vi "Leitura_pressão2CAN_temperatura.vi"() -> ()   [LabVIEW 2019]
uses:
  <vilib>/Analysis/baseanly.llb/Mean (DBL).vi
  <vilib>/Analysis/NI_AALBase.lvlib
panel:
  out "Derivada":waveform(dbl)[](graph)
  out "Tempo s":dbl
  out "Stop Press 2":bool
  in  "WindowMean":i32=20
  out "Comp Suc":sgl
  out "Error out":errorcluster {"code" format="%.0x"}
  out "Valvula Suc":sgl
  out "error out":errorcluster
  out "XY Graph 2":cluster{dbl[], dbl[]}[](graph)
  out "Stop Press":bool
  out "Stop Temp":bool
  in  "stop":bool
  out "Zerar Temp":bool
  out "Zerar Press":bool
  in  "Zerar":bool
  out "Corpo [ºC]":dbl
  out "Descarga [ºC]":dbl
  out "Reservatório [ºC]":dbl
  out "Sucção [ºC]":dbl
  out "Intermed":dbl format="%0.4f"
  out "Descarga A0":dbl format="%0.4f"
  out "Sucção A1":dbl format="%0.4f"
  out "XY Graph":cluster{dbl[], dbl[]}[](graph)
  out "Descarga/Sucção":dbl
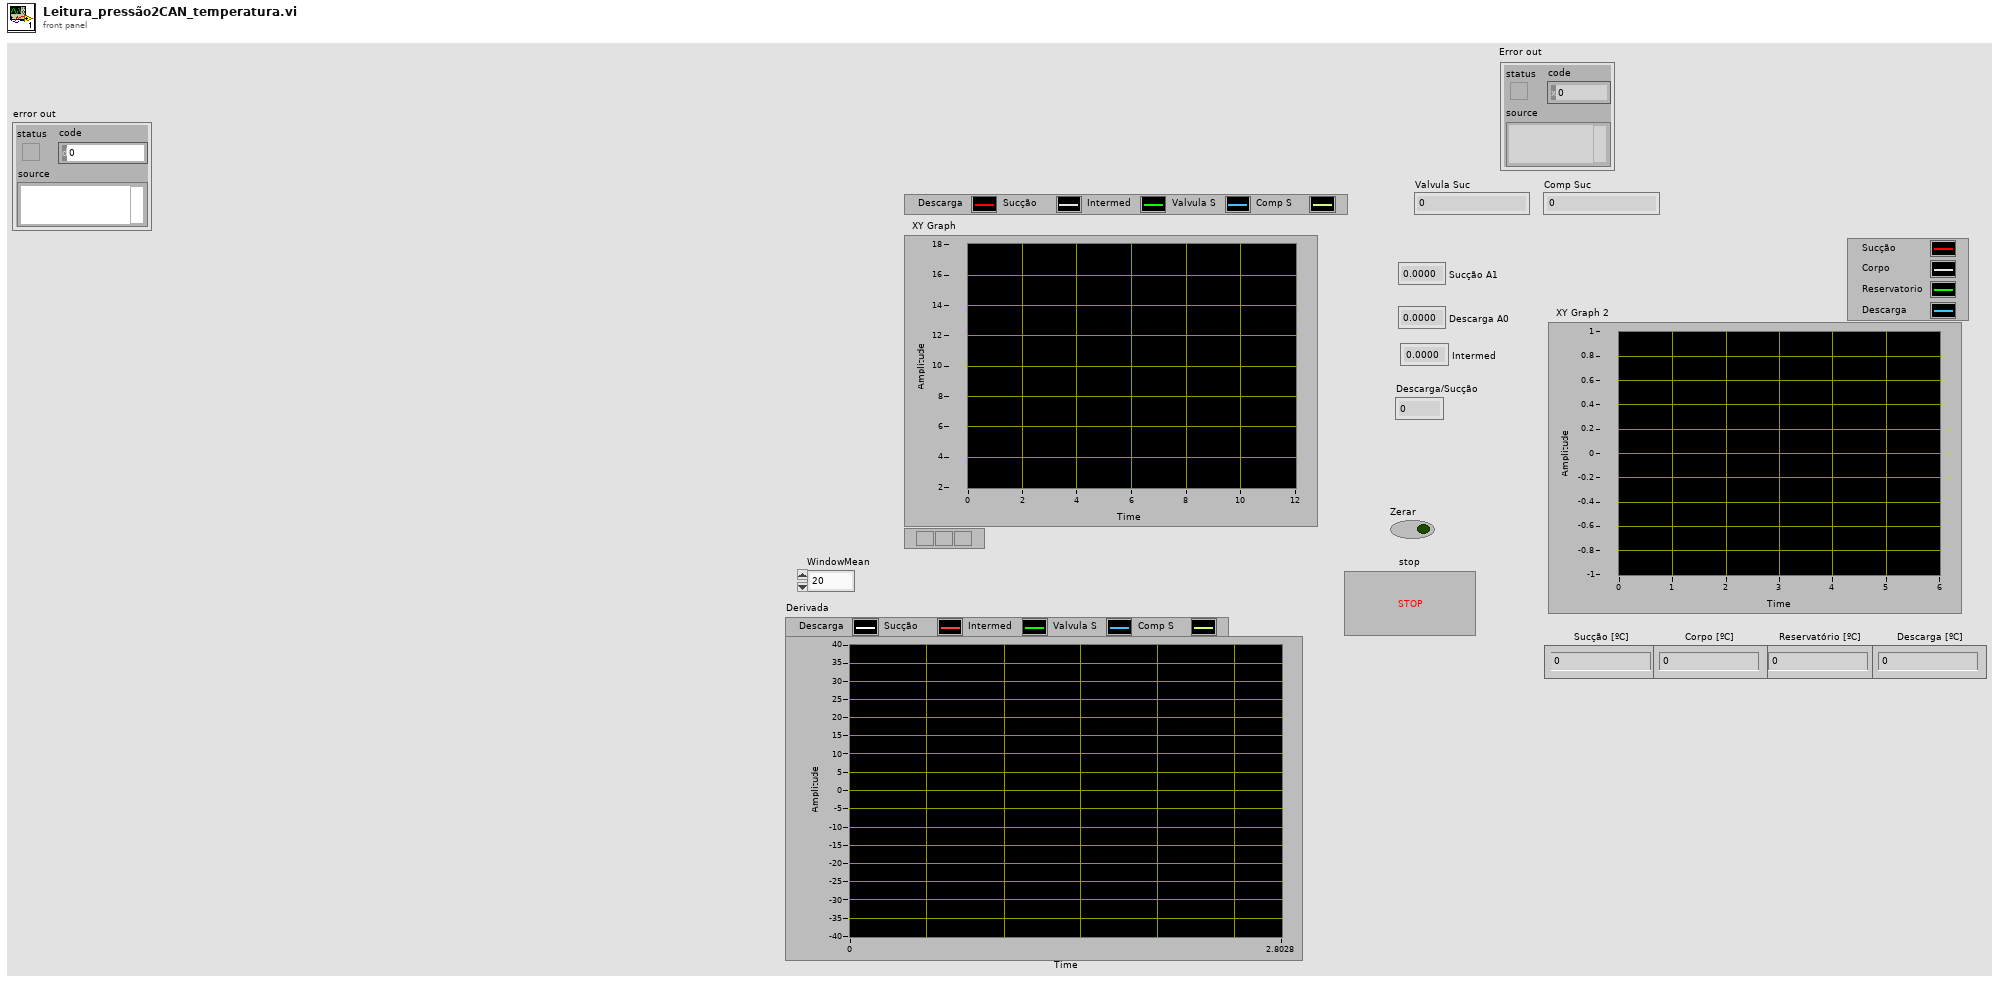
[diagram p1: front panel]
types:
  T1 = enum16{"start remote node", "stop remote node", "reset node", "reset communication", "enter preoperational"}
  T2 = typedef "xobjhandle.ctl" = u32
  T3 = enum16{"big-endian, network order", "native, host order", "little-endian"}
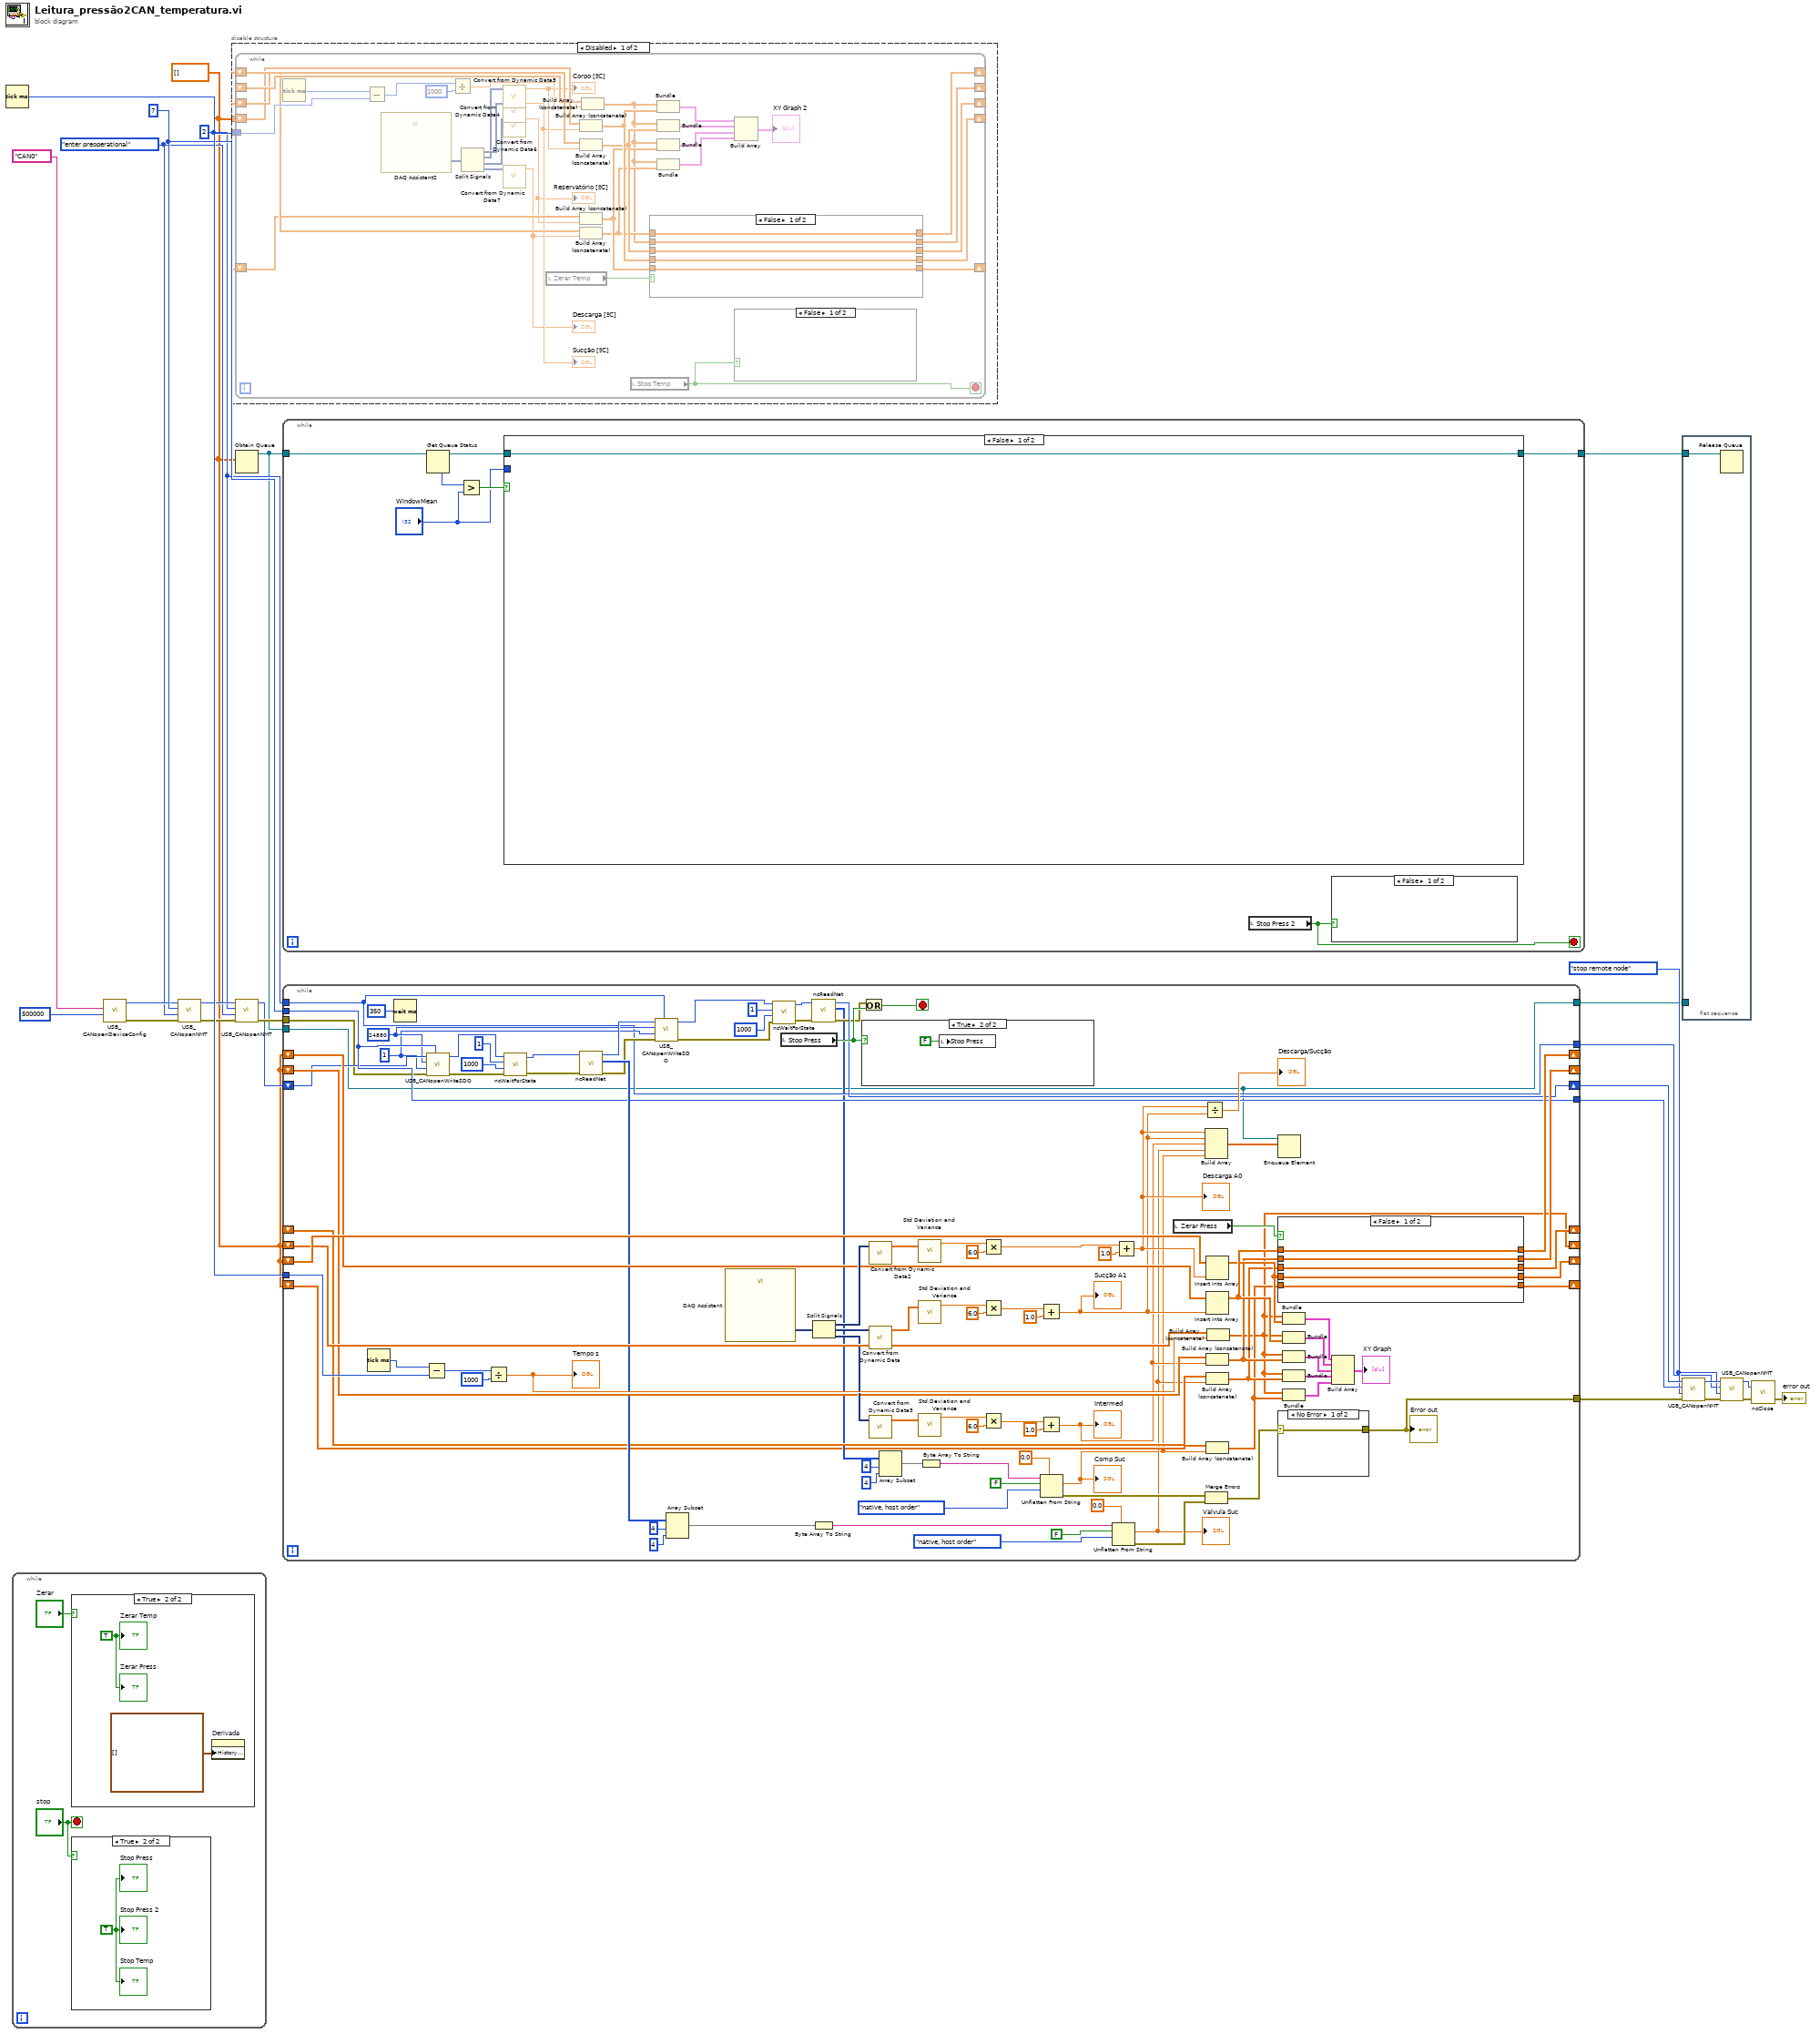
[diagram p0: block diagram]
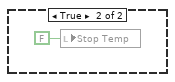
[diagram p2: hidden frame]
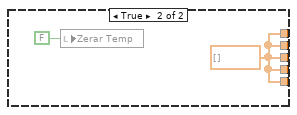
[diagram p3: hidden frame]
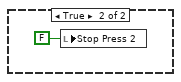
[diagram p5: hidden frame]
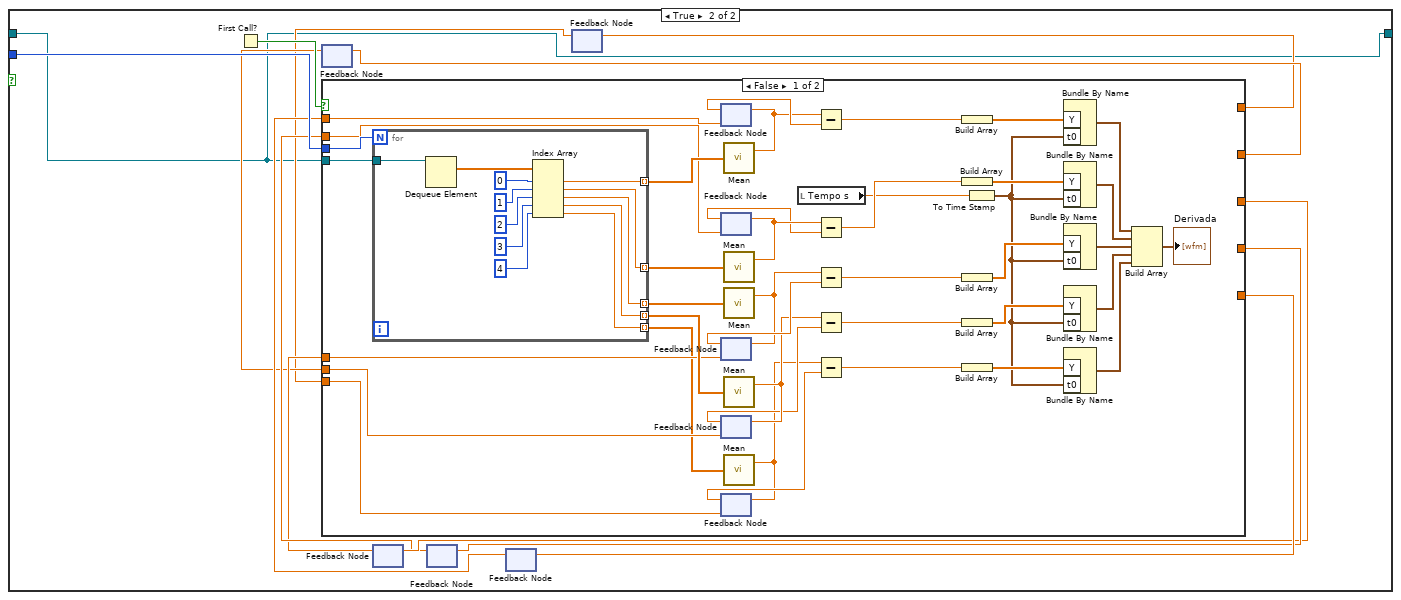
[diagram p6: hidden frame]
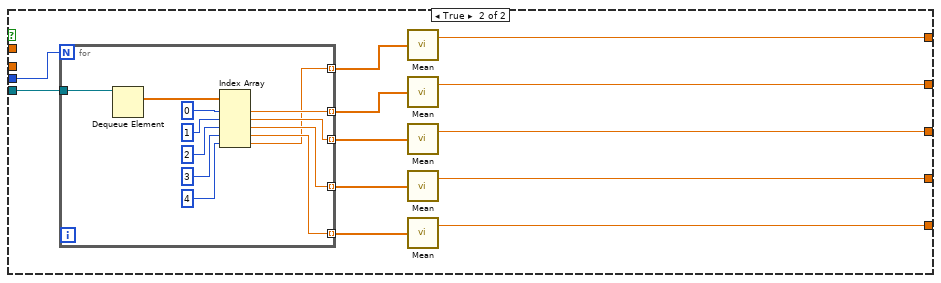
[diagram p7: hidden frame]
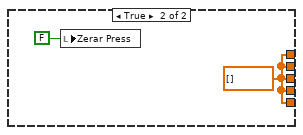
[diagram p12: hidden frame]
diagram:
  w11 = 2
  w12 = T1."enter preoperational" ("Mode")
  w21 = u32 7 ("milliseconds to wait")
  w6 = T1."stop remote node" ("Mode")
  w5 = dbl[] []
  n1 = Tick Count (ms)() -> (millisecond timer value=w26:u32)
  n2 = while {
    stop <- "stop" stop-if-true
    n3 = case shown="True" "Zerar" {
      frame False {
      }
      frame True {
        w31 = TRUE
        n4 = property on="Derivada" class="WFChart (strict)"("History Data"=waveform(dbl)[][] []) -> ()  [unwired: 2 in, 2 out]
        "Zerar Press" <- w31
        "Zerar Temp" <- w31
      }
    }
    n5 = case shown="True" "stop" {
      frame False {
      }
      frame True {
        w29 = TRUE
        "Stop Press" <- w29
        "Stop Temp" <- w29
        "Stop Press 2" <- w29
      }
    }
  }
  n6 = call "USB_CANopenDeviceConfig.vi"("Baudrate"=u32 500000, "Interface"="CAN0") -> ("Error out"=w18:errorcluster, "ObjHandle out"=w17:T2)  [unwired: 8 in]
  n7 = call "USB_CANopenNMT.vi"("error in"=w18, "Mode"=w12, "Node ID"=w21, "ObjHandle in"=w17) -> ("error out"=w15:errorcluster, "ObjHandle out"=w16:T2)  [unwired: 2 in]
  n8 = disable-structure shown="Disabled" {
    disable-tunnel: w26 -> [w33 _]
    disable-tunnel: w5 -> [w32 _]
    frame Disabled {
      n9 = while {
        tunnel: w33 -> [w62]
        shift-right: [w51] -> _
        shift-left: w32 -> [w50]
        shift-right: [w53] -> _
        shift-left: w32 -> [w52]
        shift-right: [w55] -> _
        shift-left: w32 -> [w54]
        shift-right: [w57] -> _
        shift-left: w32 -> [w56]
        shift-right: [w58] -> _
        shift-left: _ -> [w60]
        stop <- w39 stop-if-true
        n10 = Tick Count (ms)() -> (millisecond timer value=w63:u32)
        n11 = Subtract(x=w63, y=w62) -> (x-y=w64:u32)
        n12 = call "DAQ Assistant2"() -> ("data"=w69:dynamicdata)  [unwired: 17 in, 2 out]
        n13 = Divide(x=w64, y=u32 1000) -> (x/y=w59:dbl)
        n14 = Split Signals(w69) -> (w68:dynamicdata, w67:dynamicdata, w66:dynamicdata, w65:dynamicdata)  [unwired: 4 in]
        n15 = call "Convert from Dynamic Data5"("Dynamic Data Type"=w67) -> ("Scalar"=w48:dbl)  [unwired: 3 in]
        "Corpo [ºC]" <- w48
        n16 = call "Convert from Dynamic Data4"("Dynamic Data Type"=w68) -> ("Scalar"=w49:dbl)  [unwired: 3 in]
        "Sucção [ºC]" <- w49
        n17 = call "Convert from Dynamic Data6"("Dynamic Data Type"=w66) -> ("Scalar"=w47:dbl)  [unwired: 3 in]
        "Reservatório [ºC]" <- w47
        n18 = call "Convert from Dynamic Data7"("Dynamic Data Type"=w65) -> ("Scalar"=w46:dbl)  [unwired: 3 in]
        "Descarga [ºC]" <- w46
        n19 = local read "Zerar Temp"() -> (w40:bool)
        n20 = Build Array (concatenate)(w50, w49) -> (w45:dbl[])
        n21 = Build Array (concatenate)(w52, w48) -> (w44:dbl[])
        n22 = Build Array (concatenate)(w54, w47) -> (w43:dbl[])
        n23 = Build Array (concatenate)(w56, w46) -> (w42:dbl[])
        n24 = Build Array (concatenate)(w60, w59) -> (w41:dbl[])
        n25 = local read "Stop Temp"() -> (w39:bool)
        n26 = case shown="False" w40 {
          tunnel: w41 -> [w75 _]
          tunnel: [w75 w76] -> w58
          tunnel: w42 -> [w74 _]
          tunnel: [w74 w76] -> w57
          tunnel: w43 -> [w73 _]
          tunnel: [w73 w76] -> w55
          tunnel: w44 -> [w72 _]
          tunnel: [w72 w76] -> w53
          tunnel: w45 -> [w71 _]
          tunnel: [w71 w76] -> w51
          frame False {
          }
          frame True {
            w76 = dbl[] []
            n27 = local write "Zerar Temp"(FALSE ("Zerar Temp")) -> ()
          }
        }
        n28 = Bundle(w41, w45) -> (w37:cluster{dbl[], dbl[]})  [unwired: 1 in]
        n29 = Bundle(w41, w44) -> (w36:cluster{dbl[], dbl[]})  [unwired: 1 in]
        n30 = Bundle(w41, w43) -> (w35:cluster{dbl[], dbl[]})  [unwired: 1 in]
        n31 = Bundle(w41, w42) -> (w34:cluster{dbl[], dbl[]})  [unwired: 1 in]
        n32 = Build Array(w37, w36, w35, w34) -> (→"XY Graph 2":cluster{dbl[], dbl[]}[])
        n33 = case shown="False" w39 {
          frame False {
          }
          frame True {
            n34 = local write "Stop Temp"(FALSE ("Stop Temp")) -> ()
          }
        }
      }
    }
    frame Enabled {
    }
  }
  n35 = Obtain Queue(element data type=w5) -> (queue out=w4:refnum<queue>)  [unwired: 4 in, 2 out]
  n36 = call "USB_CANopenNMT.vi"("error in"=w15, "Mode"=w12, "Node ID"=w11, "ObjHandle in"=w16) -> ("error out"=w14:errorcluster, "ObjHandle out"=w13:T2)  [unwired: 2 in]
  n37 = while {
    tunnel: w4 -> [w84]
    tunnel: [w78] -> w3
    stop <- w79 stop-if-true
    n38 = Get Queue Status(queue=w84) -> (queue out=w80:refnum<queue>, # elements in queue=w83:i32)  [unwired: 2 in, 6 out]
    n39 = Greater?(x=w83, y="WindowMean") -> (0:w82:bool)
    n40 = case shown="False" w82 {
      tunnel: "WindowMean" -> [_ w99]
      tunnel: w80 -> [w86 w87]
      tunnel: [w86 w87] -> w78
      frame False {
      }
      frame True {
        n41 = First Call?() -> (First Call?: T/F=w98:bool)
        n42 = feedback #1() -> (w90:dbl)  [unwired: 1 in]
        n43 = feedback #2() -> (w91:dbl)  [unwired: 1 in]
        n44 = feedback #3() -> (w92:dbl)  [unwired: 1 in]
        n45 = feedback #4() -> (w93:dbl)  [unwired: 1 in]
        n46 = feedback #5() -> (w88:dbl)  [unwired: 1 in]
        n47 = case shown="False" w98 {
          tunnel: w99 -> [w139 w154]
          tunnel: w87 -> [w138 w159]
          tunnel: [_ w158] -> w94
          tunnel: [_ w157] -> w95
          tunnel: [_ w156] -> w96
          tunnel: [_ w155] -> w97
          tunnel: w93 -> [w125 _]
          tunnel: w92 -> [w124 _]
          tunnel: w91 -> [w123 _]
          tunnel: w90 -> [w122 _]
          tunnel: [_ w152] -> w89
          tunnel: w88 -> [w118 _]
          frame False {
            n48 = for {
              N: w139 -> [_]
              tunnel: w138 -> [w151]
              tunnel: [w145] -> w135 mode=indexing
              tunnel: [w144] -> w128 mode=indexing
              tunnel: [w143] -> w127 mode=indexing
              tunnel: [w142] -> w126 mode=indexing
              tunnel: [w140] -> w119 mode=indexing
              n49 = Dequeue Element(queue=w151) -> (element=w150:dbl[])  [unwired: 2 in, 3 out]
              n50 = Index Array(array=w150, index #1=0 ("index"), index #2=1 ("index"), index #3=2 ("index"), index #4=3 ("index"), index #5=4 ("index")) -> (element #1=w145:dbl, element #2=w144:dbl, element #3=w143:dbl, element #4=w142:dbl, element #5=w140:dbl)
            }
            n51 = feedback #6(w125) -> (w137:dbl)
            n52 = feedback #7(w124) -> (w133:dbl)
            n53 = feedback #8(w123) -> (w132:dbl)
            n54 = feedback #9(w122) -> (w129:dbl)
            n55 = feedback #10(w118) -> (w121:dbl)
            n56 = call-poly <vilib>:"Mean.vi"("X"=w135) -> ("mean"=w136:dbl)  [unwired: 1 out]
            n57 = feedback-in #6(w136) -> ()
            n58 = call-poly <vilib>:"Mean.vi"("X"=w128) -> ("mean"=w134:dbl)  [unwired: 1 out]
            n59 = feedback-in #7(w134) -> ()
            n60 = call-poly <vilib>:"Mean.vi"("X"=w127) -> ("mean"=w131:dbl)  [unwired: 1 out]
            n61 = feedback-in #8(w131) -> ()
            n62 = call-poly <vilib>:"Mean.vi"("X"=w126) -> ("mean"=w130:dbl)  [unwired: 1 out]
            n63 = feedback-in #9(w130) -> ()
            n64 = call-poly <vilib>:"Mean.vi"("X"=w119) -> ("mean"=w120:dbl)  [unwired: 1 out]
            n65 = feedback-in #10(w120) -> ()
            n66 = local read "Tempo s"() -> (w102:dbl)
            n67 = Subtract(x=w136, y=w137) -> (x-y=w116:dbl)
            n68 = Subtract(x=w134, y=w133) -> (x-y=w115:dbl)
            n69 = Subtract(x=w131, y=w132) -> (x-y=w114:dbl)
            n70 = Subtract(x=w130, y=w129) -> (x-y=w113:dbl)
            n71 = Subtract(x=w120, y=w121) -> (x-y=w112:dbl)
            n72 = Build Array(w116) -> (w117:dbl[])
            n73 = Build Array(w115) -> (w111:dbl[])
            n74 = Build Array(w114) -> (w110:dbl[])
            n75 = Build Array(w113) -> (w109:dbl[])
            n76 = Build Array(w112) -> (w108:dbl[])
            n77 = To Time Stamp(1:w102) -> (0:w101:timestamp)
            n78 = Bundle By Name("Y"=w117, "t0"=w101) -> (w107:waveform(dbl))  [unwired: 1 in]
            n79 = Bundle By Name("Y"=w111, "t0"=w101) -> (w106:waveform(dbl))  [unwired: 1 in]
            n80 = Bundle By Name("Y"=w110, "t0"=w101) -> (w105:waveform(dbl))  [unwired: 1 in]
            n81 = Bundle By Name("Y"=w109, "t0"=w101) -> (w104:waveform(dbl))  [unwired: 1 in]
            n82 = Bundle By Name("Y"=w108, "t0"=w101) -> (w103:waveform(dbl))  [unwired: 1 in]
            n83 = Build Array(w107, w106, w105, w104, w103) -> (→"Derivada":waveform(dbl)[])
          }
          frame True {
            n84 = for {
              N: w154 -> [_]
              tunnel: w159 -> [w175]
              tunnel: [w169] -> w160 mode=indexing
              tunnel: [w168] -> w161 mode=indexing
              tunnel: [w167] -> w162 mode=indexing
              tunnel: [w166] -> w163 mode=indexing
              tunnel: [w164] -> w153 mode=indexing
              n85 = Dequeue Element(queue=w175) -> (element=w174:dbl[])  [unwired: 2 in, 3 out]
              n86 = Index Array(array=w174, index #1=0 ("index"), index #2=1 ("index"), index #3=2 ("index"), index #4=3 ("index"), index #5=4 ("index")) -> (element #1=w169:dbl, element #2=w168:dbl, element #3=w167:dbl, element #4=w166:dbl, element #5=w164:dbl)
            }
            n87 = call-poly <vilib>:"Mean.vi"("X"=w153) -> ("mean"=w152:dbl)  [unwired: 1 out]
            n88 = call-poly <vilib>:"Mean.vi"("X"=w160) -> ("mean"=w158:dbl)  [unwired: 1 out]
            n89 = call-poly <vilib>:"Mean.vi"("X"=w161) -> ("mean"=w157:dbl)  [unwired: 1 out]
            n90 = call-poly <vilib>:"Mean.vi"("X"=w162) -> ("mean"=w156:dbl)  [unwired: 1 out]
            n91 = call-poly <vilib>:"Mean.vi"("X"=w163) -> ("mean"=w155:dbl)  [unwired: 1 out]
          }
        }
        n92 = feedback-in #1(w94) -> ()
        n93 = feedback-in #2(w95) -> ()
        n94 = feedback-in #3(w96) -> ()
        n95 = feedback-in #4(w97) -> ()
        n96 = feedback-in #5(w89) -> ()
      }
    }
    n97 = local read "Stop Press 2"() -> (w79:bool)
    n98 = case shown="False" w79 {
      frame False {
      }
      frame True {
        n99 = local write "Stop Press 2"(FALSE ("Stop Press")) -> ()
      }
    }
  }
  n100 = while {
    shift-right: [w263] -> _
    shift-left: w5 -> [w271]
    shift-right: [w264] -> _
    shift-left: w5 -> [w270]
    shift-right: [w183] -> _
    shift-left: w5 -> [w256]
    tunnel: w26 -> [w247]
    shift-right: [w237] -> _
    shift-left: w5 -> [w239]
    tunnel: [w226] -> w24
    tunnel: [w227] -> w23
    tunnel: w21 -> [w227]
    shift-right: [w201] -> w22
    shift-left: w13 -> [w219]
    tunnel: w14 -> [w218]
    shift-right: [w214] -> _
    shift-left: _ -> [w217]
    tunnel: w11 -> [w200]
    tunnel: [w200] -> w2
    shift-right: [w184] -> _
    shift-left: w5 -> [w187]
    tunnel: w4 -> [w176]
    tunnel: [w176] -> w1
    stop <- w204 stop-if-true
    w202 = u8 1 ("Sub Index")
    w203 = u16 24880 ("Index")
    n101 = Tick Count (ms)() -> (millisecond timer value=w249:u32)
    n102 = Wait (ms)(milliseconds to wait=u32 350) -> ()  [unwired: 1 out]
    n103 = Subtract(x=w249, y=w247) -> (x-y=w248:u32)
    n104 = call "USB_CANopenWriteSDO.vi"("Node ID"=w227, "error in"=w218, "Sub Index"=w202, "Index"=w203, "ObjHandle in"=w219) -> ("error out"=w221:errorcluster, "ObjHandle out"=w223:T2)  [unwired: 5 in]
    n105 = Divide(x=w248, y=u32 1000) -> (x/y=w250:dbl)
    "Tempo s" <- w250
    n106 = call <vilib>:"ncWaitForState.vi"("Error in"=w221, "Timeout"=u32 1000, "DesiredState"=u32 1, "ObjHandle in"=w223) -> ("Error out"=w220:errorcluster, "ObjHandle out"=w222:T2)  [unwired: 1 out]
    n107 = call <vilib>:"ncReadNet.vi"("ObjHandle in"=w222, "Error in"=w220) -> ("ObjHandle out"=w207:T2, "Data"=w228:u8[], "Error out"=w206:errorcluster)  [unwired: 2 in, 4 out]
    n108 = call "USB_CANopenWriteSDO.vi"("Node ID"=w200, "error in"=w206, "Sub Index"=w202, "Index"=w203, "ObjHandle in"=w207) -> ("error out"=w212:errorcluster, "ObjHandle out"=w210:T2)  [unwired: 5 in]
    n109 = Array Subset(array=w228, index=4, length=4) -> (w229:u8[])
    n110 = call "DAQ Assistant"() -> ("data"=w276:dynamicdata)  [unwired: 17 in, 2 out]
    n111 = call <vilib>:"ncWaitForState.vi"("Error in"=w212, "Timeout"=u32 1000, "DesiredState"=u32 1, "ObjHandle in"=w210) -> ("Error out"=w213:errorcluster, "ObjHandle out"=w211:T2)  [unwired: 1 out]
    n112 = local read "Stop Press"() -> (w205:bool)
    n113 = call <vilib>:"ncReadNet.vi"("ObjHandle in"=w211, "Error in"=w213) -> ("ObjHandle out"=w201:T2, "Data"=w193:u8[], "Error out"=w198:errorcluster)  [unwired: 2 in, 4 out]
    n114 = Byte Array To String(unsigned byte array=w229) -> (string=w235:string)
    n115 = Split Signals(w276) -> (w274:dynamicdata, w275:dynamicdata, w246:dynamicdata)  [unwired: 3 in]
    n116 = case shown="True" w205 {
      frame False {
      }
      frame True {
        n117 = local write "Stop Press"(FALSE ("Stop Press")) -> ()
      }
    }
    n118 = Or(x=w198, y=w205) -> (x .or. y?=w204:bool)
    n119 = call "Convert from Dynamic Data2"("Dynamic Data Type"=w274) -> ("Array"=w273:dbl[])  [unwired: 3 in]
    n120 = call "Convert from Dynamic Data"("Dynamic Data Type"=w275) -> ("Array"=w272:dbl[])  [unwired: 3 in]
    n121 = call "Convert from Dynamic Data3"("Dynamic Data Type"=w246) -> ("Array"=w245:dbl[])  [unwired: 3 in]
    n122 = Array Subset(array=w193, index=4, length=4) -> (w196:u8[])
    n123 = call <vilib>:"Std Deviation and Variance.vi"("X"=w273) -> ("mean"=w268:dbl)  [unwired: 1 in, 2 out]
    n124 = call <vilib>:"Std Deviation and Variance.vi"("X"=w272) -> ("mean"=w266:dbl)  [unwired: 1 in, 2 out]
    n125 = call <vilib>:"Std Deviation and Variance.vi"("X"=w245) -> ("mean"=w241:dbl)  [unwired: 1 in, 2 out]
    n126 = Byte Array To String(unsigned byte array=w196) -> (string=w189:string)
    n127 = Multiply(x=w268, y=6.0) -> (x*y=w259:dbl)
    n128 = Multiply(x=w266, y=6.0) -> (x*y=w260:dbl)
    n129 = Multiply(x=w241, y=6.0) -> (x*y=w244:dbl)
    n130 = Add(x=w260, y=1.0) -> (x+y=w181:dbl)
    "Sucção A1" <- w181
    n131 = Add(x=w244, y=1.0) -> (x+y=w180:dbl)
    "Intermed" <- w180
    n132 = Unflatten From String(type=sgl 0.0, binary string=w189, data includes array or string size? (T)=FALSE, byte order (0:big-endian, network order)=T3."native, host order") -> (value=w178:sgl, error out=w188:errorcluster)  [unwired: 1 in, 1 out]
    "Comp Suc" <- w178
    n133 = Unflatten From String(type=sgl 0.0, binary string=w235, data includes array or string size? (T)=FALSE, byte order (0:big-endian, network order)=T3."native, host order") -> (value=w179:sgl, error out=w199:errorcluster)  [unwired: 1 in, 1 out]
    "Valvula Suc" <- w179
    n134 = Add(x=w259, y=1.0) -> (x+y=w182:dbl)
    "Descarga A0" <- w182
    n135 = local read "Zerar Press"() -> (w236:bool)
    n136 = Divide(x=w182, y=w181) -> (x/y=→"Descarga/Sucção":dbl)
    n137 = Build Array(w182, w181, w180, w179, w178) -> (w177:dbl[])
    n138 = Merge Errors(w188, w199) -> (w197:errorcluster)
    n139 = Insert Into Array(array=w271, new element=w182) -> (w254:dbl[])  [unwired: 1 in]
    n140 = Insert Into Array(array=w270, new element=w181) -> (w255:dbl[])  [unwired: 1 in]
    n141 = Build Array (concatenate)(w239, w180) -> (w238:dbl[])
    n142 = Build Array (concatenate)(w217, w179) -> (w215:dbl[])
    n143 = Build Array (concatenate)(w187, w178) -> (w185:dbl[])
    n144 = Build Array (concatenate)(w256, w250) -> (w183:dbl[])
    n145 = Enqueue Element(queue=w176, element=w177) -> ()  [unwired: 2 in, 3 out]
    n146 = case shown="False" w236 {
      tunnel: w255 -> [w283 _]
      tunnel: [w283 w284] -> w264
      tunnel: w254 -> [w282 _]
      tunnel: [w282 w284] -> w263
      tunnel: w238 -> [w281 _]
      tunnel: [w281 w284] -> w237
      tunnel: w215 -> [w280 _]
      tunnel: [w280 w284] -> w214
      tunnel: w185 -> [w279 _]
      tunnel: [w279 w284] -> w184
      frame False {
      }
      frame True {
        w284 = dbl[] []
        n147 = local write "Zerar Press"(FALSE ("Zerar Temp")) -> ()
      }
    }
    n148 = case shown="No Error" w197 {
      selector: w197 -> [w277 _]
      tunnel: [w277 _] -> w226
      frame No Error {
      }
      frame Error {
      }
    }
    "Error out" <- w226
    n149 = Bundle(w183, w254) -> (w253:cluster{dbl[], dbl[]})  [unwired: 1 in]
    n150 = Bundle(w183, w255) -> (w252:cluster{dbl[], dbl[]})  [unwired: 1 in]
    n151 = Bundle(w183, w238) -> (w240:cluster{dbl[], dbl[]})  [unwired: 1 in]
    n152 = Bundle(w183, w215) -> (w216:cluster{dbl[], dbl[]})  [unwired: 1 in]
    n153 = Bundle(w183, w185) -> (w186:cluster{dbl[], dbl[]})  [unwired: 1 in]
    n154 = Build Array(w253, w252, w240, w216, w186) -> (→"XY Graph":cluster{dbl[], dbl[]}[])
  }
  n155 = flat-sequence {
    tunnel: w3 -> [w286]
    tunnel: w1 -> [_]
    frame #0 {
      n156 = Release Queue(queue=w286) -> ()  [unwired: 2 in, 3 out]
    }
  }
  n157 = call "USB_CANopenNMT.vi"("error in"=w24, "Mode"=w6, "Node ID"=w23, "ObjHandle in"=w22) -> ("error out"=w8:errorcluster, "ObjHandle out"=w7:T2)  [unwired: 2 in]
  n158 = call "USB_CANopenNMT.vi"("error in"=w8, "Mode"=w6, "Node ID"=w2, "ObjHandle in"=w7) -> ("error out"=w9:errorcluster, "ObjHandle out"=w10:T2)  [unwired: 2 in]
  n159 = call <vilib>:"ncClose.vi"("Error in"=w9, "ObjHandle in"=w10) -> ("Error out"=→"error out":errorcluster)  [unwired: 1 in]
